vi "Write Report.vi"(8 "error in (no error)":errorcluster, 10 "Resource In":variant, 11 "Analyze Results Energy in":refnum<class "Analyze Results Energy.lvclass">) -> (0 "error out":errorcluster, 2 "Resource Out":variant, 3 "Analyze Results Energy out":refnum<class "Analyze Results Energy.lvclass">)   [LabVIEW 2014, in "Analyze Results Energy.lvclass"]
uses:
  Analyze Results Energy.lvclass
  <vilib>/Utility/config.llb/Config Data RefNum.ctl
  Results Base/Analyze Results Base.lvclass/Analyze Results Base.ctl
  Analyze Results Energy.lvclass/Analyze Results Energy.ctl
  Results Base/Read Section.vi
  <vilib>/Utility/config.llb/Write Key (Double).vi
  Results Total Counts/Analyze Results Total Counts.lvclass
  <vilib>/Utility/config.llb/NI_LVConfig.lvlib
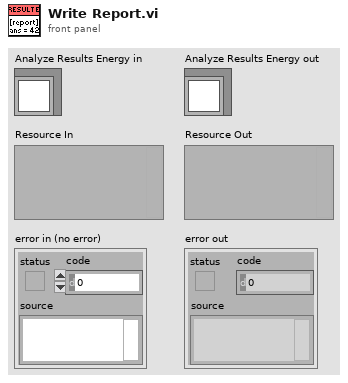
[diagram p1: front panel]
types:
  T1 = typedef "NI_LVConfig.lvlib/Config Data RefNum.ctl" = refnum<k1>
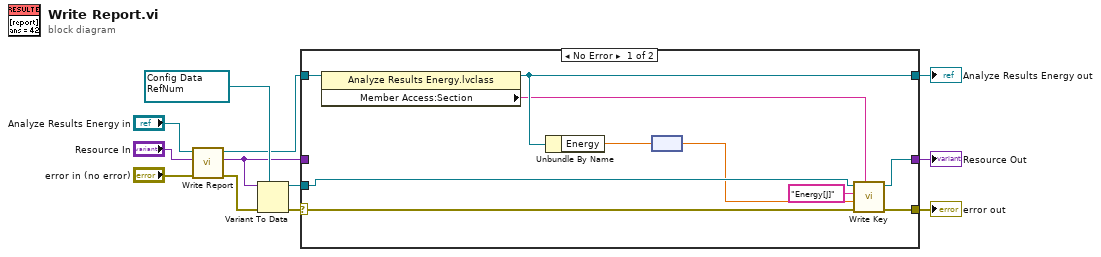
[diagram p0: block diagram]
diagram:
  w9 = T1 refnum items=["config data"] ("refnum")
  n1 = call-parent "Write Report.vi"("error in (no error)"="error in (no error)", "Resource In"="Resource In", "Analyze Results Total Counts in"="Analyze Results Energy in") -> ("error out"=w6:errorcluster, "Resource Out"=w5:variant, "Analyze Results Total Counts out"=w4:refnum<class "Analyze Results Energy.lvclass">)  [unwired: 6 in]
  n2 = Variant To Data(error in=w6, type=w9, Variant=w5) -> (data=w8:T1, error out=w7:errorcluster)
  n3 = case shown="No Error" w7 {
    selector: w7 -> [w19 w24]
    tunnel: w8 -> [w20 _]
    tunnel: w4 -> [w22 w23]
    tunnel: [w21 w23] -> w3
    tunnel: [w17 w25] -> w2
    tunnel: [w16 w24] -> w1
    tunnel: w5 -> [_ w25]
    frame No Error {
      n4 = property class="Analyze Results Energy.lvclass"(reference=w22) -> (reference out=w21:refnum<class "Analyze Results Energy.lvclass">, "Member Access:Section"=w18:string)  [unwired: 1 in, 1 out]
      n5 = Unbundle By Name(w21) -> ("Energy"=w15:dbl[unit])
      n6 = node(w15) -> (w14:dbl)
      n7 = call-poly <vilib>:"Write Key.vi"("section"=w18, "error in (no error)"=w19, "value"=w14, "key"="Energy[J]", "refnum"=w20) -> ("error out"=w16:errorcluster, "refnum out"=w17:T1)  [unwired: 4 in, 1 out]
    }
    frame Error {
    }
  }
  "error out" <- w1
  "Analyze Results Energy out" <- w3
  "Resource Out" <- w2
